vi "Initialize.vi"(7 "Serial Configuration":T1={"Baud Rate"=9600, "Parity"=0, "Data Bits"=8, "Flow Control"=4} {"Flow Control" items=["None", "XON/XOFF", "RTS/CTS", "XON/XOFF & RTS/CTS", "DTR/DSR", "XON/XOFF & DTR/DSR"]; "Data Bits" items=["7"=7, "8"=8]; "Parity" items=["None", "Odd", "Even", "Mark", "Space"]; "Baud Rate" items=["300"=300, "600"=600, "1200"=1200, "2400"=2400, "4800"=4800, "9600"=9600, "19200"=19200]}, 8 "error in (no error)":errorcluster, 9 "Reset (True)":bool=TRUE, 10 "ID Query (True)":bool=TRUE, 11 "VISA resource name":refnum<visa-resource-name>) -> (0 "error out":errorcluster, 3 "VISA resource name out":refnum<visa-resource-name>)   [LabVIEW 2012, in "Agilent 33XXX Series.lvlib"]
doc: "Establishes communication with the instrument and optionally performs an instrument identification query and/or an instrument reset. It also places the instrument in a default state needed for other instrument driver operations. Therefore, call this VI before calling other instrument driver VIs for this instrument. Generally, you need to call the <B>Initialize VI</B> only once at the beginning of an application."
uses:
  Agilent 33XXX Series.lvlib
panel:
  # "(c) 2005- 2013 National Instruments.  ALL RIGHTS RESERVED."
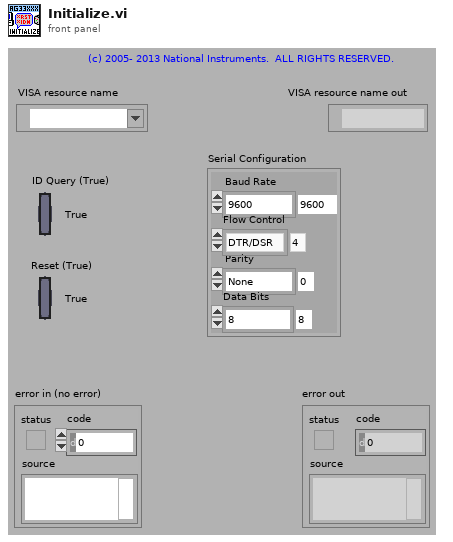
[diagram p1: front panel]
types:
  T1 = cluster{"Baud Rate":u32, "Parity":u16, "Data Bits":u16, "Flow Control":u16}
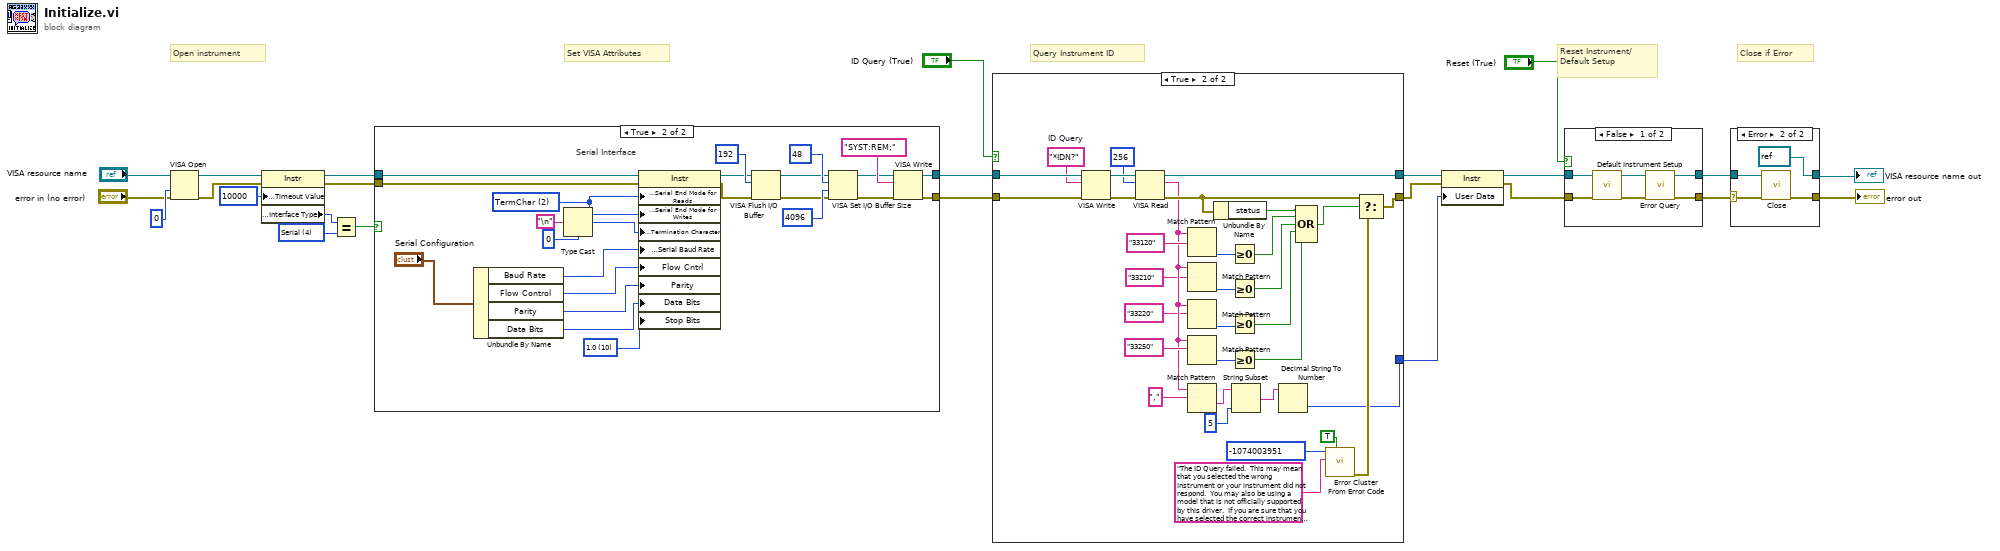
[diagram p0: block diagram]
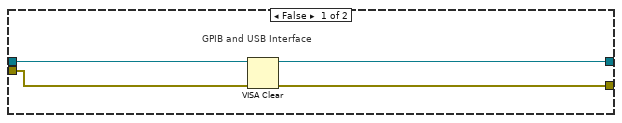
[diagram p2: hidden frame]
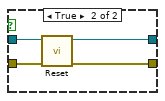
[diagram p4: hidden frame]
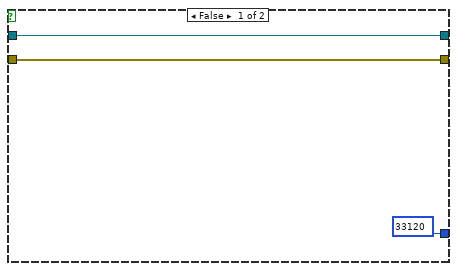
[diagram p5: hidden frame]
diagram:
  w17 = u16 4 items=["GPIB"=1, "VXI"=2, "GPIB-VXI"=3, "Serial"=4, "PXI"=5, "TCPIP"=6, "USB"=7] ("Interface Information:Interface Type")
  # "Set VISA Attributes"
  # "Close if Error"
  # "Query Instrument ID"
  # "Reset Instrument/\nDefault Setup"
  # "Open instrument"
  n1 = VISA Open(access mode=u32 0, error in (no error)="error in (no error)", VISA resource name="VISA resource name") -> (VISA resource name=w14:refnum<visa-resource-name>, error out=w13:errorcluster)  [unwired: 2 in]
  n2 = property class="Instr"(reference=w14, error in=w13, "General Settings:Timeout Value"=u32 10000) -> (reference out=w20:refnum<visa-resource-name>, error out=w19:errorcluster, "Interface Information:Interface Type"=w24:u16)
  n3 = Equal?(x=w24, y=w17) -> (x = y?=w18:bool)
  n4 = case shown="True" w18 {
    tunnel: [w26 w40] -> w22
    tunnel: [w25 w41] -> w21
    tunnel: w20 -> [w28 w51]
    tunnel: w19 -> [w27 w52]
    frame False {
      # "GPIB and USB Interface"
      n5 = VISA Clear(VISA resource name=w28, error in (no error)=w27) -> (VISA resource name out=w26:refnum<visa-resource-name>, error out=w25:errorcluster)
    }
    frame True {
      w30 = u16 10 items=["1.0"=10, "1.5"=15, "2.0"=20] ("Serial Settings:Stop Bits")
      w48 = u16 2 items=["None", "LastBit", "TermChar"] ("Serial Settings:Serial End Mode for Reads")
      # "Serial Interface"
      n6 = Unbundle By Name("Serial Configuration") -> ("Baud Rate"=w45:u32, "Flow Control"=w29:u16, "Parity"=w44:u16, "Data Bits"=w43:u16)
      n7 = Type Cast(type=u8 0, x="\n" ("Line Feed Constant")) -> (*(type *) &x=w47:u8)
      n8 = property class="Instr"(reference=w51, error in=w52, "Serial Settings:Serial End Mode for Reads"=w48, "Serial Settings:Serial End Mode for Writes"=w48, "Message Based Settings:Termination Character"=w47, "Serial Settings:Serial Baud Rate"=w45, "Flow Cntrl"=w29, "Parity"=w44, "Data Bits"=w43, "Stop Bits"=w30) -> (reference out=w38:refnum<visa-resource-name>, error out=w37:errorcluster)
      n9 = VISA Flush I/O Buffer(VISA resource name=w38, mask (16)=u16 192, error in (no error)=w37) -> (VISA resource name out=w33:refnum<visa-resource-name>, error out=w34:errorcluster)
      n10 = VISA Set I/O Buffer Size(VISA resource name=w33, mask (16)=u16 48, size (4096)=u32 4096 ("size (0)"), error in (no error)=w34) -> (VISA resource name out=w32:refnum<visa-resource-name>, error out=w31:errorcluster)
      n11 = VISA Write(VISA resource name=w32, write buffer="SYST:REM;", error in (no error)=w31) -> (VISA resource name out=w40:refnum<visa-resource-name>, error out=w41:errorcluster)  [unwired: 1 out]
    }
  }
  n12 = case shown="True" "ID Query (True)" {
    tunnel: [w54 w88] -> w11
    tunnel: [w55 w85] -> w12
    tunnel: w22 -> [w55 w86]
    tunnel: w21 -> [w54 w87]
    tunnel: [33120 w69] -> w8
    frame False {
    }
    frame True {
      w80 = "*IDN?"  # ID Query
      n13 = VISA Write(VISA resource name=w86, write buffer=w80, error in (no error)=w87) -> (VISA resource name out=w84:refnum<visa-resource-name>, error out=w83:errorcluster)  [unwired: 1 out]
      n14 = VISA Read(VISA resource name=w84, byte count=u32 256, error in (no error)=w83) -> (VISA resource name out=w85:refnum<visa-resource-name>, read buffer=w61:string, error out=w68:errorcluster)  [unwired: 1 out]
      n15 = Match Pattern(string=w61, regular expression="33120") -> (offset past match=w82:i32)  [unwired: 1 in, 3 out]
      n16 = Match Pattern(string=w61, regular expression="33210") -> (offset past match=w62:i32)  [unwired: 1 in, 3 out]
      n17 = Match Pattern(string=w61, regular expression="33220") -> (offset past match=w60:i32)  [unwired: 1 in, 3 out]
      n18 = Match Pattern(string=w61, regular expression="33250") -> (offset past match=w65:i32)  [unwired: 1 in, 3 out]
      n19 = Match Pattern(string=w61, regular expression=",") -> (after substring=w71:string)  [unwired: 1 in, 3 out]
      n20 = Unbundle By Name(w68) -> ("status"=w67:bool)
      n21 = Greater Or Equal To 0?(x=w82) -> (x >= 0?=w66:bool)
      n22 = Greater Or Equal To 0?(x=w62) -> (x >= 0?=w64:bool)
      n23 = Greater Or Equal To 0?(x=w60) -> (x >= 0?=w59:bool)
      n24 = Greater Or Equal To 0?(x=w65) -> (x >= 0?=w58:bool)
      n25 = String Subset(string=w71, length (rest)=5 ("length (rest)")) -> (substring=w72:string)  [unwired: 1 in]
      n26 = Decimal String To Number(string=w72) -> (number=w69:i32)  [unwired: 2 in, 1 out]
      n27 = Compound Arithmetic op=OR(w67, w66, w64, w59, w58) -> (w63:bool)
      n28 = call <vilib>:"Error Cluster From Error Code.vi"("show call chain? (False)"=TRUE, "error message (\"\")"="The ID Query failed.  This may mean that you selected the wrong instrument or your instrument did not respond.  You may also be using a model that is not officially supported by this driver.  If you are sure that you have selected the correct instrument and it is responding, try disabling the ID Query." ("Source (VI Name)"), "error code (0)"=-1074003951 ("Code")) -> ("error out"=w79:errorcluster)  [unwired: 6 in]
      n29 = Select(t=w68, s=w63, f=w79) -> (s? t:f=w88:errorcluster)
    }
  }
  n30 = property class="Instr"(reference=w12, error in=w11, "User Data"=w8) -> (reference out=w9:refnum<visa-resource-name>, error out=w10:errorcluster)
  n31 = case shown="False" "Reset (True)" {
    tunnel: w10 -> [w93 w95]
    tunnel: [w89 w98] -> w15
    tunnel: w9 -> [w94 w96]
    tunnel: [w90 w97] -> w16
    frame False {
      n32 = call "Default Instrument Setup.vi"("error in (no error)"=w93, "VISA resource name"=w94) -> ("error out"=w91:errorcluster, "VISA resource name out"=w92:refnum<visa-resource-name>)  [unwired: 8 in]
      n33 = call "Error Query.vi"("error in (no error)"=w91, "VISA resource name"=w92) -> ("error out"=w89:errorcluster, "VISA resource name out"=w90:refnum<visa-resource-name>)  [unwired: 6 in, 2 out]
    }
    frame True {
      n34 = call "Reset.vi"("error in (no error)"=w95, "VISA resource name"=w96) -> ("error out"=w98:errorcluster, "VISA resource name out"=w97:refnum<visa-resource-name>)  [unwired: 8 in]
    }
  }
  n35 = case shown="Error" w15 {
    selector: w15 -> [w99 w102]
    tunnel: w16 -> [w100 w103]
    tunnel: [w100 refnum<visa-resource-name> refnum ("VISA resource name out")] -> w5
    tunnel: [w99 w104] -> w4
    frame No Error {
    }
    frame Error {
      n36 = call "Close.vi"("error in (no error)"=w102, "VISA resource name"=w103) -> ("error out"=w104:errorcluster)  [unwired: 9 in]
    }
  }
  "VISA resource name out" <- w5
  "error out" <- w4
